vi "insert hi score.vi"(8 "Error In":errorcluster, 10 "Score to Insert":T1, 11 "Score Array In":T1[](array[typedef])) -> (0 "Error Out":errorcluster, 2 "Lowest Score Out":dbl, 3 "Score Array Out":T1[](array[typedef]))   [LabVIEW 2017]
uses:
  controls/scores.ctl
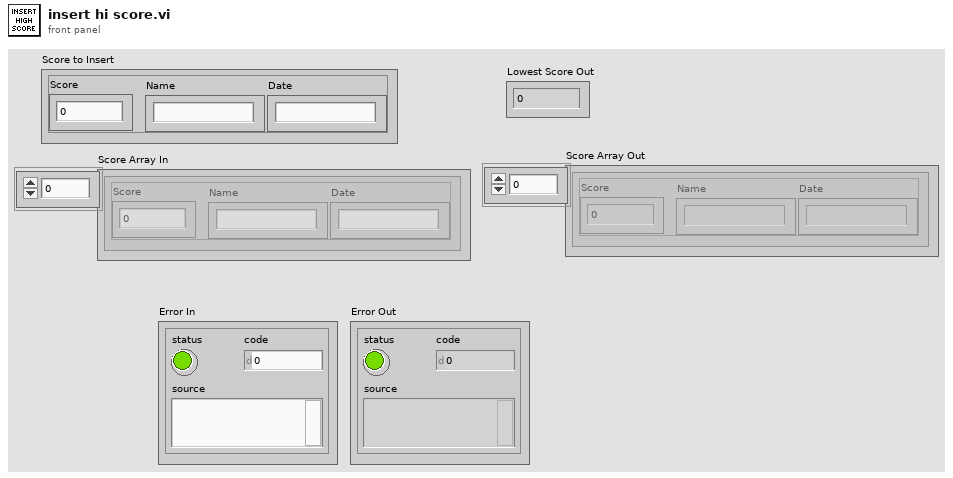
[diagram p1: front panel]
types:
  T1 = typedef "scores.ctl" = cluster{"Score":dbl, "Name":string, "Date":string}
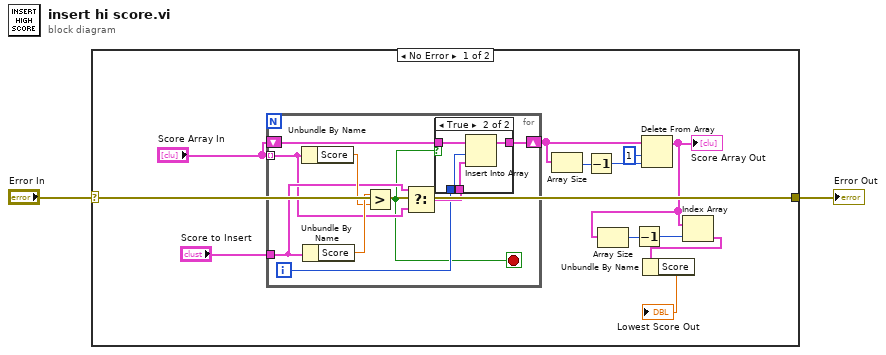
[diagram p0: block diagram]
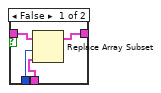
[diagram p2: hidden frame]
diagram:
  n1 = case shown="No Error" "Error In" {
    selector: "Error In" -> [w9 w32]
    tunnel: [w9 w32] -> w1
    frame No Error {
      n2 = for {
        tunnel: "Score Array In" -> [w18] mode=indexing
        shift-right: [w20] -> w11
        shift-left: "Score Array In" -> [w21]
        tunnel: "Score to Insert" -> [w19]
        i -> [w16]
        stop <- w15 stop-if-true
        n3 = Unbundle By Name(w18) -> ("Score"=w22:dbl)
        n4 = Unbundle By Name(w19) -> ("Score"=w23:dbl)
        n5 = Greater?(x=w23, y=w22) -> (0:w15:bool)
        n6 = Select(t=w19, s=w15, f=w18) -> (s? t:f=w17:T1)
        n7 = case shown="True" w15 {
          tunnel: w21 -> [w27 w31]
          tunnel: [w24 w30] -> w20
          tunnel: w17 -> [w25 w29]
          tunnel: w16 -> [w26 w28]
          frame False {
            n8 = Replace Array Subset(array=w27, new element=w25, index=w26) -> (w24:T1[])
          }
          frame True {
            n9 = Insert Into Array(array=w31, index=w28, new element=w29) -> (w30:T1[])
          }
        }
      }
      n10 = Array Size(array=w11) -> (size(s)=w12:i32)
      n11 = Decrement(x=w12) -> (x-1=w8:i32)
      n12 = Delete From Array(array=w11, length=1, index=w8) -> (array with subset deleted=w3:T1[])  [unwired: 1 out]
      "Score Array Out" <- w3
      n13 = Array Size(array=w3) -> (size(s)=w5:i32)
      n14 = Decrement(x=w5) -> (x-1=w4:i32)
      n15 = Index Array(array=w3, index=w4) -> (element=w7:T1)
      n16 = Unbundle By Name(w7) -> ("Score"=→"Lowest Score Out":dbl)
    }
    frame Error {
    }
  }
  "Error Out" <- w1
